vi "Add Randomness.vi"(8 "Amplitude\n(default 1)":dbl=1.0, 11 "Numeric in":dbl) -> (3 "Numeric out":dbl)   [LabVIEW 2011]
doc: "Adds random noise to the input signal, with the noise ranging from -amplitude to +amplitude. If no input signal is provided, returns just the noise."
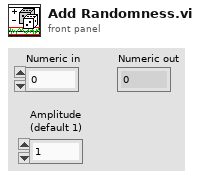
[diagram p1: front panel]
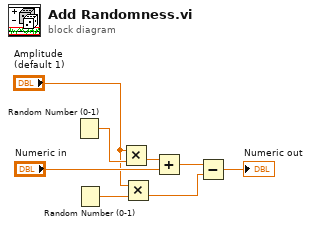
[diagram p0: block diagram]
diagram:
  n1 = Random Number (0-1)() -> (number: 0 to 1=w7:dbl)
  n2 = Random Number (0-1)() -> (number: 0 to 1=w8:dbl)
  n3 = Multiply(x="Amplitude\n(default 1)", y=w7) -> (x*y=w3:dbl)
  n4 = Multiply(x="Amplitude\n(default 1)", y=w8) -> (x*y=w2:dbl)
  n5 = Add(x=w3, y="Numeric in") -> (x+y=w5:dbl)
  n6 = Subtract(x=w5, y=w2) -> (x-y=→"Numeric out":dbl)
